vi "iclExeIsRunning.vi"(8 "error in":errorcluster, 11 "iclWasAlreadyRunning":bool) -> (0 "error out":errorcluster)   [LabVIEW 2023, in "horiba.lvlib" / "DeviceManager.lvlib"]
doc: "This broadcast is sent when the ICL has been launched or a already running ICL has been detected.\n_____\nCreated using DQMH Event Scripter 7.0.1.1316."
uses:
  DeviceManager.lvlib
  iclStarted Argument--cluster.ctl
panel:
  # "Connector Pane"
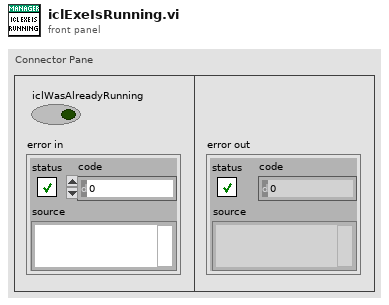
[diagram p1: front panel]
types:
  T1 = typedef "horiba.lvlib/DeviceManager.lvlib/iclStarted Argument--cluster.ctl" = cluster{"iclIsRunning":bool}
  T2 = typedef "horiba.lvlib/DeviceManager.lvlib/Broadcast Events--cluster.ctl" = cluster{"Module Did Init":refnum<user-event>, "Status Updated":refnum<user-event>, "Error Reported":refnum<user-event>, "Module Did Stop":refnum<user-event>, "Update Module Execution Status":refnum<user-event>, "iclIsRunning":refnum<user-event>, "websocketConnectionOpened":refnum<user-event>, "devicesDiscovered":refnum<user-event>}
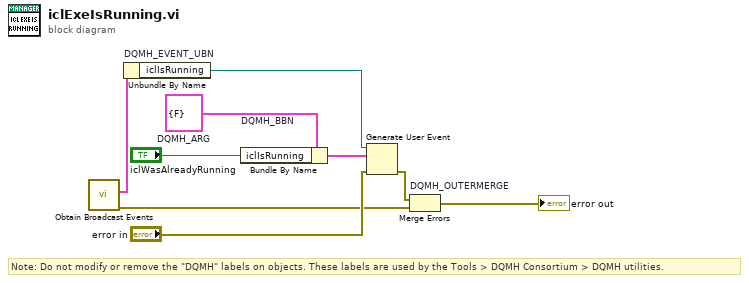
[diagram p0: block diagram]
diagram:
  w4 = T1 {"iclIsRunning"=FALSE}  # DQMH_ARG
  # "Note: Do not modify or remove the \"DQMH\" labels on objects. These labels are used by the Tools > DQMH Consortium > DQMH utilities."
  n1 = call "Obtain Broadcast Events.vi"() -> ("error out"=w3:errorcluster, "DeviceManager Broadcast Events"=w2:T2)  [unwired: 10 in]
  n2 = Unbundle By Name "DQMH_EVENT_UBN"(w2) -> ("iclIsRunning"=w6:refnum<user-event>)
  n3 = Bundle By Name "DQMH_BBN"(cluster=w4, "iclIsRunning"="iclWasAlreadyRunning") -> (w7:T1)
  n4 = Generate User Event(user event=w6, event data cluster=w7, error in="error in") -> (error out=w5:errorcluster)  [unwired: 1 in, 1 out]
  n5 = Merge Errors "DQMH_OUTERMERGE"(w5, w3) -> (→"error out":errorcluster)
